vi "onMarkAsChanged.vi"(8 "error in (no error)":errorcluster, 9 "keys":string[](array[string]), 10 "Qualified Name":string, 11 "ConfigManager.Text in":refnum<class "ConfigManager.Text.lvclass">) -> (0 "error out":errorcluster, 3 "ConfigManager.Text out":refnum<class "ConfigManager.Text.lvclass">)   [LabVIEW 2013, in "CfgManager.Text.lvlib" / "ConfigManager.Text.lvclass"]
uses:
  ConfigManager.Text.lvclass
  payload -- cluster.ctl
  Response - cluster.ctl
  ConfigManager.Text.lvclass/ConfigManager.Text.ctl
  <vilib>/Utility/error.llb/Clear Errors.vi
  <vilib>/LabVIEW Open Source Project/Unicity/Delimiter/Delimiter.lvclass
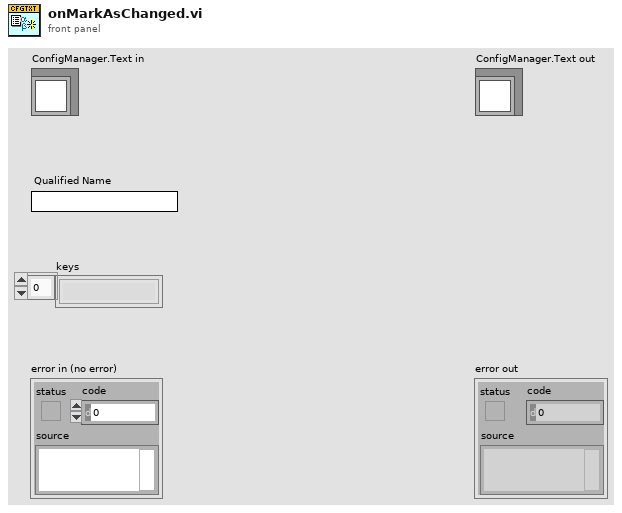
[diagram p1: front panel]
types:
  T1 = typedef "CfgManager.Text.lvlib/ConfigManager.Text.lvclass/payload -- cluster.ctl" = cluster{"command":string, "args":variant, "query":refnum<notifier>, "ack":refnum<notifier>}
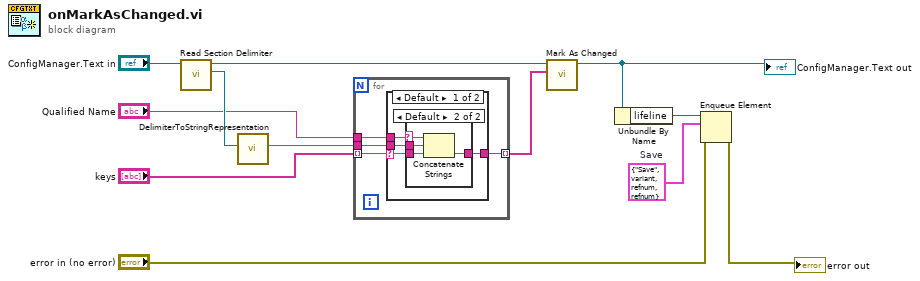
[diagram p0: block diagram]
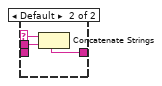
[diagram p4: hidden frame]
diagram:
  w3 = T1 {"command"="Save", "args"=variant, "query"=refnum, "ack"=refnum}  # Save
  n1 = call "Read Section Delimiter.vi"("ConfigManager.Text in"="ConfigManager.Text in") -> ("Section Delimiter"=w12:refnum<class "Delimiter.lvclass">, "ConfigManager.Text out"=w6:refnum<class "ConfigManager.Text.lvclass">)  [unwired: 9 in]
  n2 = call <vilib>:"DelimiterToStringRepresentation.vi"("Delimiter"=w12) -> ("String representation"=w11:string)  [unwired: 10 in]
  n3 = for {
    tunnel: w11 -> [w16]
    tunnel: "Qualified Name" -> [w15]
    tunnel: "keys" -> [w14] mode=indexing
    tunnel: [w13] -> w8 mode=indexing
    n4 = case shown="Default" w14 {
      selector: w14 -> [w17 w26]
      tunnel: w15 -> [w20 w29]
      tunnel: w16 -> [w19 w28]
      tunnel: [w18 w27] -> w13
      frame Default {
        n5 = case shown="Default" w20 {
          selector: w20 -> [_ w22]
          tunnel: w17 -> [w21 w25]
          tunnel: [w21 w24] -> w18
          tunnel: w19 -> [_ w23]
          frame "" {
          }
          frame Default {
            n6 = Concatenate Strings(w22, w23, w25) -> (w24:string)
          }
        }
      }
      frame "" {
        n7 = case shown="\"\"" w29 {
          selector: w29 -> [_ w30]
          tunnel: w26 -> [_ _]
          tunnel: [_ w32] -> w27
          tunnel: w28 -> [_ w31]
          frame "" {
          }
          frame Default {
            n8 = Concatenate Strings(w30, w31) -> (w32:string)
          }
        }
      }
    }
  }
  n9 = call "Mark As Changed.vi"("Changed elements"=w8, "ConfigManager.Text in"=w6) -> ("ConfigManager.Text out"=w5:refnum<class "ConfigManager.Text.lvclass">)  [unwired: 9 in]
  "ConfigManager.Text out" <- w5
  n10 = Unbundle By Name(w5) -> ("lifeline"=w4:refnum<queue>)
  n11 = Enqueue Element(queue=w4, element=w3, error in (no error)="error in (no error)") -> (error out=→"error out":errorcluster)  [unwired: 1 in, 2 out]
